vi "Create New VI.vi"(10 "Open Frontpanel":bool, 11 "Data Cluster in":T1) -> (1 "message":string, 2 "ID":i32, 3 "Data Cluster out":T1)   [LabVIEW 2025, in "Scripting Server.lvlib"]
uses:
  Scripting Server.lvlib
  Module Data--cluster.ctl
  <vilib>/Utility/error.llb/DialogType.ctl
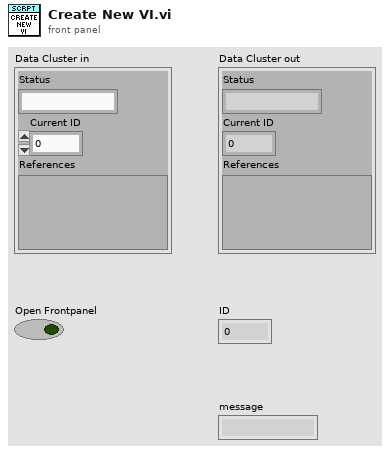
[diagram p1: front panel]
types:
  T1 = typedef "Scripting Server.lvlib/Module Data--cluster.ctl" = cluster{"Status":string, "Current ID":i32, "References":variant}
  T2 = typedef "DialogType.ctl" = u16
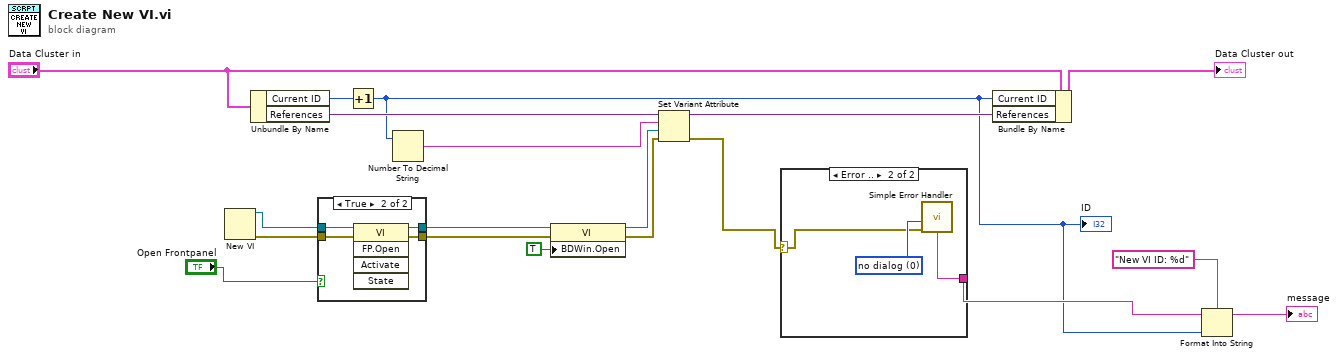
[diagram p0: block diagram]
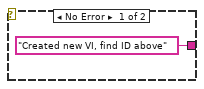
[diagram p2: hidden frame]
diagram:
  n1 = New VI() -> (0:w10:errorcluster, 3:w5:refnum<vi>)  [unwired: 7 in]
  n2 = Unbundle By Name("Data Cluster in") -> ("Current ID"=w13:i32, "References"=w14:variant)
  n3 = case shown="True" "Open Frontpanel" {
    tunnel: w10 -> [w20 w25]
    tunnel: w5 -> [w21 w24]
    tunnel: [w20 w23] -> w16
    tunnel: [w21 w22] -> w3
    frame False {
    }
    frame True {
      n4 = invoke class="VI" method="FP.Open"(reference=w24, error in=w25) -> (reference out=w22:refnum<vi>, error out=w23:errorcluster)  [unwired: 3 in, 3 out]
    }
  }
  n5 = Increment(x=w13) -> (x+1=w6:i32)
  "ID" <- w6
  n6 = Number To Decimal String(number=w6) -> (decimal integer string=w18:string)  [unwired: 1 in]
  n7 = property class="VI"(reference=w3, error in=w16, "BDWin.Open"=TRUE ("Block Diagram Window:Open")) -> (reference out=w2:refnum<vi>, error out=w4:errorcluster)
  n8 = Set Variant Attribute(Variant=w14, name=w18, value=w2, error in=w4) -> (Variant out=w15:variant, error out=w9:errorcluster)  [unwired: 1 out]
  n9 = case shown="Error .." w9 {
    selector: w9 -> [_ w27]
    tunnel: ["Created new VI, find ID above" ("message") w29] -> w17
    frame No Error {
    }
    frame Error {
      w28 = T2 0 items=["no dialog", "OK message", "continue or stop message", "OK message + warnings", "continue/stop + warnings"] ("type of dialog (OK msg:1)")
      n10 = call <vilib>:"Simple Error Handler.vi"("type of dialog (OK msg:1)"=w28, "error in (no error)"=w27) -> ("message"=w29:string)  [unwired: 3 in, 4 out]
    }
  }
  n11 = Bundle By Name(cluster="Data Cluster in", "Current ID"=w6, "References"=w15) -> (→"Data Cluster out":T1)
  n12 = Format Into String(format string="New VI ID: %d", initial string=w17, w6) -> (resulting string=→"message":string)  [unwired: 1 in, 1 out]
